vi "testRecursiveCompoundStructure.vi"(8 "error in (no error)":errorcluster, 11 "TestCase in":refnum<class "EasyXMLTest.lvclass">) -> (0 "error out":errorcluster, 3 "TestCase out":refnum<class "EasyXMLTest.lvclass">)   [LabVIEW 2011, in "EasyXMLTest.lvclass"]
doc: "Verify that error in is not overwritten"
uses:
  EasyXMLTest.lvclass
panel:
  out "Produced Data":variant
  out "Input Data":variant
  out "XML String":string
  out "Generated XML String":string
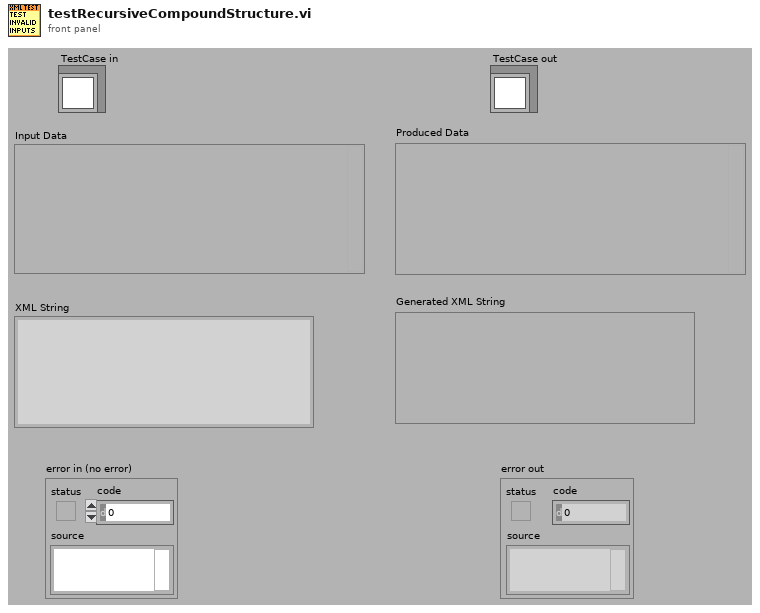
[diagram p1: front panel]
types:
  T1 = cluster{"my boolean":bool, "my dbl":dbl, "my array":cluster{"my boolean":bool, "my dbl":dbl}[], "my array 2":cluster{"my boolean":bool, "my dbl":dbl}[], "my cluster":cluster{"my boolean":bool, "my dbl":dbl, "my array":cluster{"my boolean":bool, "my dbl":dbl}[], "my array 2":cluster{"my boolean":bool, "my dbl":dbl}[]}}
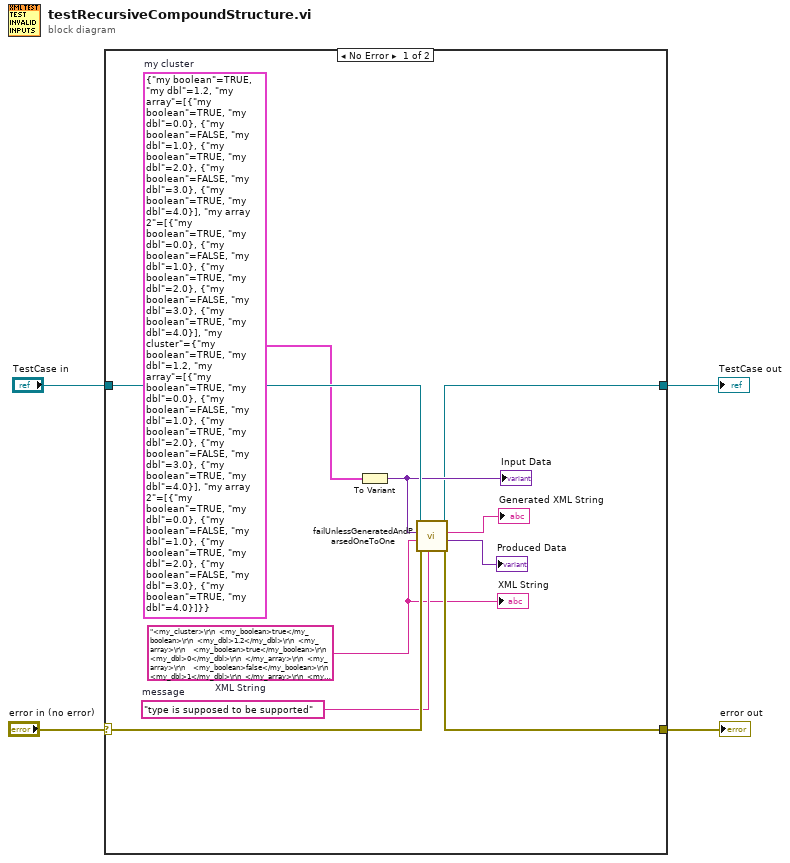
[diagram p0: block diagram]
diagram:
  n1 = case shown="No Error" "error in (no error)" {
    selector: "error in (no error)" -> [w13 w16]
    tunnel: [w8 w16] -> w2
    tunnel: [w7 w15] -> w1
    tunnel: "TestCase in" -> [w14 w15]
    frame No Error {
      w5 = T1 {"my boolean"=TRUE, "my dbl"=1.2, "my array"=[{"my boolean"=TRUE, "my dbl"=0.0}, {"my boolean"=FALSE, "my dbl"=1.0}, {"my boolean"=TRUE, "my dbl"=2.0}, {"my boolean"=FALSE, "my dbl"=3.0}, {"my boolean"=TRUE, "my dbl"=4.0}], "my array 2"=[{"my boolean"=TRUE, "my dbl"=0.0}, {"my boolean"=FALSE, "my dbl"=1.0}, {"my boolean"=TRUE, "my dbl"=2.0}, {"my boolean"=FALSE, "my dbl"=3.0}, {"my boolean"=TRUE, "my dbl"=4.0}], "my cluster"={"my boolean"=TRUE, "my dbl"=1.2, "my array"=[{"my boolean"=TRUE, "my dbl"=0.0}, {"my boolean"=FALSE, "my dbl"=1.0}, {"my boolean"=TRUE, "my dbl"=2.0}, {"my boolean"=FALSE, "my dbl"=3.0}, {"my boolean"=TRUE, "my dbl"=4.0}], "my array 2"=[{"my boolean"=TRUE, "my dbl"=0.0}, {"my boolean"=FALSE, "my dbl"=1.0}, {"my boolean"=TRUE, "my dbl"=2.0}, {"my boolean"=FALSE, "my dbl"=3.0}, {"my boolean"=TRUE, "my dbl"=4.0}]}}  # my cluster
      w6 = "<my_cluster>\r\n  <my_boolean>true</my_boolean>\r\n  <my_dbl>1.2</my_dbl>\r\n  <my_array>\r\n    <my_boolean>true</my_boolean>\r\n    <my_dbl>0</my_dbl>\r\n  </my_array>\r\n  <my_array>\r\n    <my_boolean>false</my_boolean>\r\n    <my_dbl>1</my_dbl>\r\n  </my_array>\r\n  <my_array>\r\n    <my_boolean>true</my_boolean>\r\n    <my_dbl>2</my_dbl>\r\n  </my_array>\r\n  <my_array>\r\n    <my_boolean>false</my_boolean>\r\n    <my_dbl>3</my_dbl>\r\n  </my_array>\r\n  <my_array>\r\n    <my_boolean>true</my_boolean>\r\n    <my_dbl>4</my_dbl>\r\n  </my_array>\r\n  <my_array_2>\r\n    <my_boolean>true</my_boolean>\r\n    <my_dbl>0</my_dbl>\r\n  </my_array_2>\r\n  <my_array_2>\r\n    <my_boolean>false</my_boolean>\r\n    <my_dbl>1</my_dbl>\r\n  </my_array_2>\r\n  <my_array_2>\r\n    <my_boolean>true</my_boolean>\r\n    <my_dbl>2</my_dbl>\r\n  </my_array_2>\r\n  <my_array_2>\r\n    <my_boolean>false</my_boolean>\r\n    <my_dbl>3</my_dbl>\r\n  </my_array_2>\r\n  <my_array_2>\r\n    <my_boolean>true</my_boolean>\r\n    <my_dbl>4</my_dbl>\r\n  </my_array_2>\r\n  <my_cluster>\r\n    <my_boolean>true</my_boolean>\r\n    <my_dbl>1.2</my_dbl>\r\n    <my_array>\r\n      <my_boolean>true</my_boolean>\r\n      <my_dbl>0</my_dbl>\r\n    </my_array>\r\n    <my_array>\r\n      <my_boolean>false</my_boolean>\r\n      <my_dbl>1</my_dbl>\r\n    </my_array>\r\n    <my_array>\r\n      <my_boolean>true</my_boolean>\r\n      <my_dbl>2</my_dbl>\r\n    </my_array>\r\n    <my_array>\r\n      <my_boolean>false</my_boolean>\r\n      <my_dbl>3</my_dbl>\r\n    </my_array>\r\n    <my_array>\r\n      <my_boolean>true</my_boolean>\r\n      <my_dbl>4</my_dbl>\r\n    </my_array>\r\n    <my_array_2>\r\n      <my_boolean>true</my_boolean>\r\n      <my_dbl>0</my_dbl>\r\n    </my_array_2>\r\n    <my_array_2>\r\n      <my_boolean>false</my_boolean>\r\n      <my_dbl>1</my_dbl>\r\n    </my_array_2>\r\n    <my_array_2>\r\n      <my_boolean>true</my_boolean>\r\n      <my_dbl>2</my_dbl>\r\n    </my_array_2>\r\n    <my_array_2>\r\n      <my_boolean>false</my_boolean>\r\n      <my_dbl>3</my_dbl>\r\n    </my_array_2>\r\n    <my_array_2>\r\n      <my_boolean>true</my_boolean>\r\n      <my_dbl>4</my_dbl>\r\n    </my_array_2>\r\n  </my_cluster>\r\n</my_cluster>"  # XML String
      w12 = "type is supposed to be supported"  # message
      n2 = To Variant(anything=w5) -> (Variant=w10:variant)
      "Input Data" <- w10
      n3 = call "failUnlessGeneratedAndParsedOneToOne.vi"("message (\"\")"=w12, "error in"=w13, "XML String"=w6, "Data"=w10, "EasyXMLTest in"=w14) -> ("error out"=w8:errorcluster, "Produced Data"=→"Produced Data":variant, "Generated XML String"=→"Generated XML String":string, "EasyXMLTest out"=w7:refnum<class "EasyXMLTest.lvclass">)  [unwired: 3 in]
      "XML String" <- w6
    }
    frame Error {
    }
  }
  "error out" <- w2
  "TestCase out" <- w1
